vi "Create Value - 1D Array Boolean.vi"(5 "1D Boolean":bool[](array[boolean]), 9 "Create as 1D Array?":bool=TRUE, 11 "error in (no error)":errorcluster) -> (4 "JSON Tree":variant, 15 "error out":errorcluster)   [LabVIEW 2015, in "i3-json.lvlib"]
doc: "Creates a new JSON Object of the given type"
uses:
  i3-json.lvlib
  JSON Types/JSON Type.ctl
  JSON Types/JSON Compatible Type.ctl
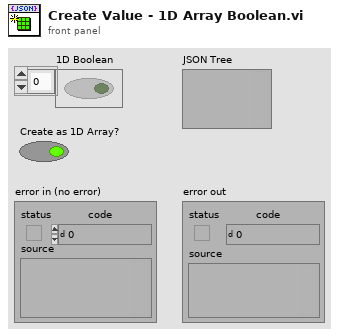
[diagram p1: front panel]
types:
  T1 = typedef "i3-json.lvlib/JSON Compatible Type.ctl" = enum16{"1D Double Array", "1D String Array", "1D Boolean Array", "Unknown"}
  T2 = typedef "i3-json.lvlib/JSON Type.ctl" = enum8{"JSON Compatible", "JSON Array", "JSON Object", "JSON Null", "Double", "String", "Boolean", "Unknown"}
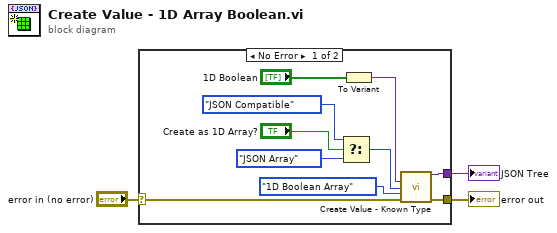
[diagram p0: block diagram]
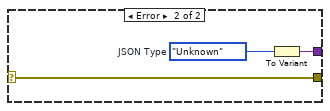
[diagram p2: hidden frame]
diagram:
  n1 = case shown="No Error" "error in (no error)" {
    selector: "error in (no error)" -> [w12 w14]
    tunnel: [w11 w14] -> w2
    tunnel: [w13 w15] -> w1
    frame No Error {
      n2 = Select(t=JSON_Type."JSON Compatible" ("JSON Type"), s="Create as 1D Array?", f=JSON_Type."JSON Array" ("JSON Type")) -> (s? t:f=w5:T2)
      n3 = To Variant(anything="1D Boolean") -> (Variant=w4:variant)
      n4 = call "Create Value - Known Type.vi"("Value"=w4, "JSON Type"=w5, "JSON Compatible Type"=JSON_Compatible_Type."1D Boolean Array", "error in (no error)"=w12) -> ("JSON Tree"=w13:variant, "error out"=w11:errorcluster)  [unwired: 10 in]
    }
    frame Error {
      w16 = JSON_Type."Unknown"  # JSON Type
      n5 = To Variant(anything=w16) -> (Variant=w15:variant)
    }
  }
  "JSON Tree" <- w1
  "error out" <- w2
